vi "CloseDevice.vi"(8 "error in":errorcluster, 11 "CmdLib In":refnum<k24>) -> (0 "error out":errorcluster, 3 "CmdLib Out":refnum<k24>)   [LabVIEW 2013]
uses:
  C:/GEECS/Developers Version/source/Device Driver/Picomotor8742dotNet/NewFocus/CmdLib.dll
  CmdLib.dll
  Global Variables.vi
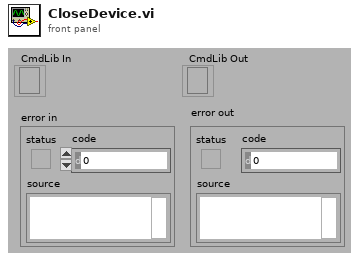
[diagram p1: front panel]
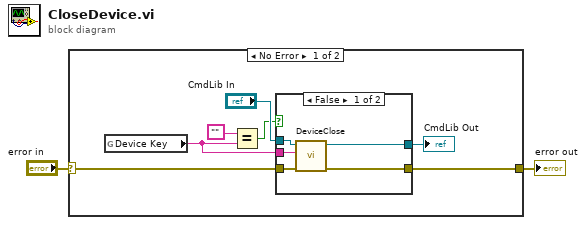
[diagram p0: block diagram]
diagram:
  n1 = case shown="No Error" "error in" {
    selector: "error in" -> [w3 w17]
    tunnel: [w7 w17] -> w2
    frame No Error {
      n2 = global read "Global Variables.vi" "Device Key"() -> (w9:string)
      n3 = Equal?(x="", y=w9) -> (x = y?=w4:bool)
      n4 = case shown="False" w4 {
        tunnel: [w14 w16] -> w6
        tunnel: [w13 w15] -> w7
        tunnel: w3 -> [w12 w15]
        tunnel: "CmdLib In" -> [w11 w16]
        tunnel: w9 -> [w10 _]
        frame False {
          n5 = call "DeviceClose.vi"("error in (no error)"=w12, "DeviceKey In"=w10, "CmdLib In"=w11) -> ("error out"=w13:errorcluster, "CmdLib Out"=w14:refnum<k24>)  [unwired: 2 in, 1 out]
        }
        frame True {
        }
      }
      "CmdLib Out" <- w6
    }
    frame Error {
    }
  }
  "error out" <- w2
